vi "Get ITL Data.vi"() -> ()   [LabVIEW 2015]
uses:
  <vilib>/Instr/_visa.llb/GPIB Status Boolean Array.ctl
  Xitron 2503AH Library.lvlib
panel:
  out "ibsta":T1
  out "data":string
  out "array":dbl[](array[numeric])
  out "String output":string
  in  "IEEE Add.":string="2"
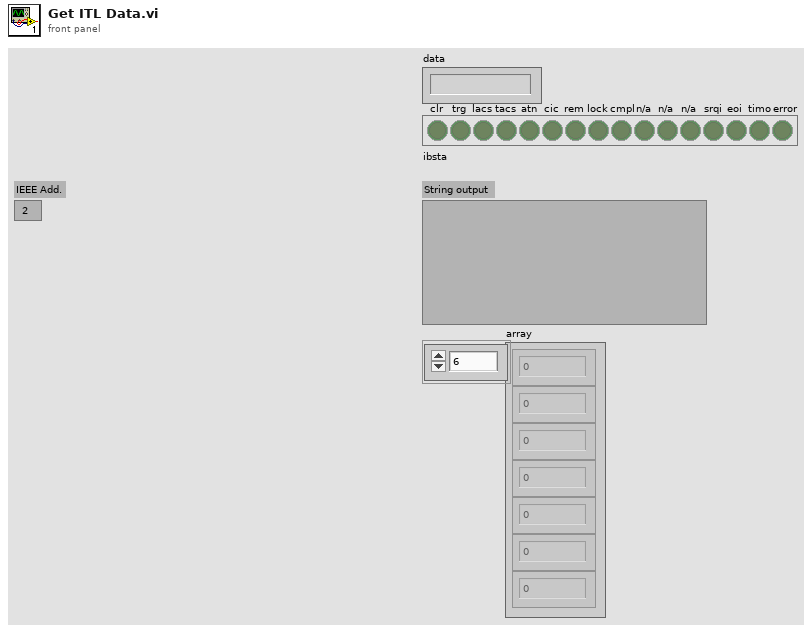
[diagram p1: front panel]
types:
  T1 = typedef "GPIB Status Boolean Array.ctl" = bool[]
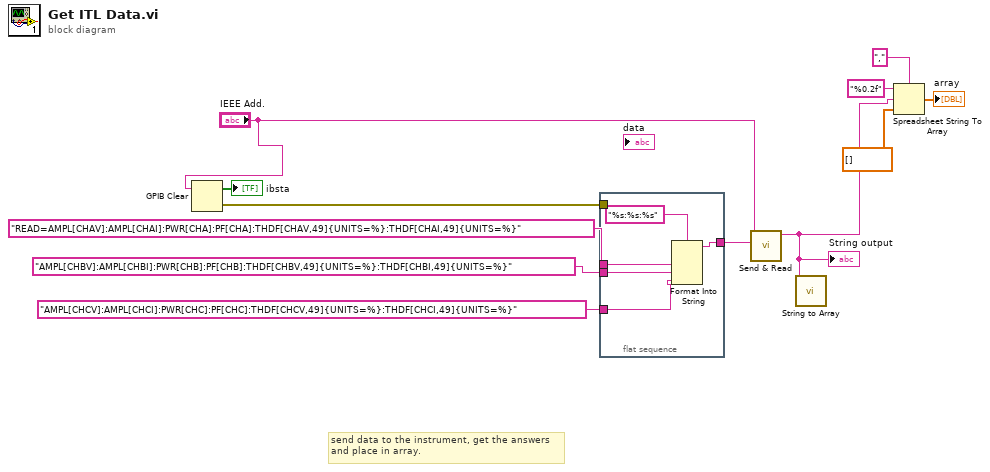
[diagram p0: block diagram]
diagram:
  # "send data to the instrument, get the answers\nand place in array."
  n1 = GPIB Clear(3:"IEEE Add.") -> (0:w1:errorcluster, 1:→"ibsta":bool[])  [unwired: 1 in]
  n2 = flat-sequence {
    tunnel: "READ=AMPL[CHAV]:AMPL[CHAI]:PWR[CHA]:PF[CHA]:THDF[CHAV,49]{UNITS=%}:THDF[CHAI,49]{UNITS=%}" -> [w16]
    tunnel: "AMPL[CHBV]:AMPL[CHBI]:PWR[CHB]:PF[CHB]:THDF[CHBV,49]{UNITS=%}:THDF[CHBI,49]{UNITS=%}" -> [w15]
    tunnel: "AMPL[CHCV]:AMPL[CHCI]:PWR[CHC]:PF[CHC]:THDF[CHCV,49]{UNITS=%}:THDF[CHCI,49]{UNITS=%}" -> [w14]
    tunnel: [w13] -> w4
    tunnel: w1 -> [_]
    frame #0 {
      n3 = Format Into String(format string="%s:%s:%s", w16, w15, w14) -> (resulting string=w13:string)  [unwired: 2 in, 1 out]
    }
  }
  n4 = call "Send & Read"("Data to be sent"=w4, "IEEE Add."="IEEE Add.") -> ("String output"=w10:string)  [unwired: 8 in, 1 out]
  "String output" <- w10
  n5 = call "String to Array"("String in"=w10) -> ()  [unwired: 10 in, 1 out]
  n6 = Spreadsheet String To Array(delimiter (Tab)=",", format string="%0.2f", spreadsheet string=w10, array type (2D Dbl)=dbl[] []) -> (array=→"array":dbl[])
